vi "Logger_SendMessage.vi"(8 "error in (no error)":errorcluster caption="错误输入（无错误）", 9 "LoggerMessage":string, 10 "LoggerCode":i32=-1, 11 "LoggerKind":enum16{"软件上传日志", "软件其他日志", "软件错误日志", "软件监控日志"}(ring)=enum."软件监控日志") -> (0 "error out":errorcluster caption="错误输出")   [LabVIEW 2019, in "Logger.lvclass"]
uses:
  <userlib>/Logger/Logger.lvclass
  <userlib>/Logger/Ctls/LoggerMessage.ctl
  <userlib>/Logger/Logger.lvclass/Logger.ctl
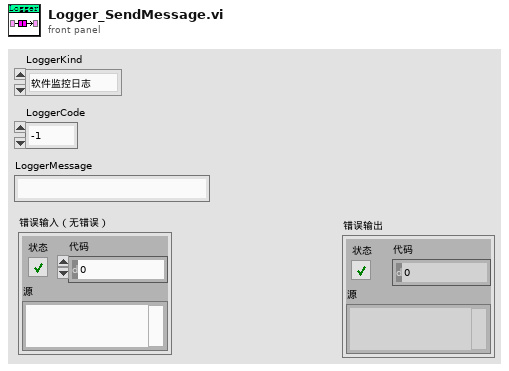
[diagram p1: front panel]
types:
  T1 = typedef "Logger.lvclass/LoggerMessage.ctl" = cluster{"LoggerKind":enum16{"软件上传日志", "软件其他日志", "软件错误日志", "软件监控日志"}, "LoggerMessage":string, "LoggerCode":i32, "LoggerCallChain":string, "LoggerTime":string}
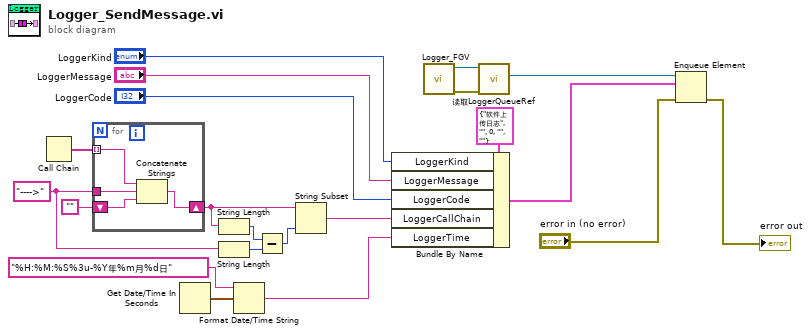
[diagram p0: block diagram]
diagram:
  w4 = "---->"
  n1 = Call Chain() -> (call chain=w17:string[])
  n2 = for {
    tunnel: w17 -> [w25] mode=indexing
    shift-right: [w22] -> w5
    shift-left: "" -> [w23]
    tunnel: w4 -> [w24]
    n3 = Concatenate Strings(w25, w24, w23) -> (w22:string)
  }
  n4 = Get Date/Time In Seconds() -> (seconds since 1Jan1904=w9:timestamp)
  n5 = String Length(string=w5) -> (length=w2:i32)
  n6 = String Length(string=w4) -> (length=w3:i32)
  n7 = Format Date/Time String(time format string (%c)="%H:%M:%S%3u-%Y年%m月%d日" ("时间格式字符串(%c)"), seconds (now)=w9) -> (date/time string=w7:string)  [unwired: 1 in]
  n8 = Subtract(x=w2, y=w3) -> (x-y=w1:i32)
  n9 = String Subset(string=w5, length (rest)=w1) -> (substring=w6:string)  [unwired: 1 in]
  n10 = Bundle By Name(cluster=T1 {"LoggerKind"=enum."软件上传日志", "LoggerMessage"="", "LoggerCode"=0, "LoggerCallChain"="", "LoggerTime"=""} ("元素"), "LoggerKind"="LoggerKind", "LoggerMessage"="LoggerMessage", "LoggerCode"="LoggerCode", "LoggerCallChain"=w6, "LoggerTime"=w7) -> (w20:T1)
  n11 = call <userlib>:"Logger_FGV.vi"() -> ("error out"=w11:errorcluster, "Logger 输出"=w12:refnum<class "Logger.lvclass">)  [unwired: 10 in]
  n12 = call "读取LoggerQueueRef.vi"("error in (no error)"=w11, "Logger输入"=w12) -> ("LoggerQueueRef"=w10:refnum<queue>)  [unwired: 7 in, 2 out]
  n13 = Enqueue Element(queue=w10, element=w20, error in (no error)="error in (no error)") -> (error out=→"error out":errorcluster)  [unwired: 1 in, 2 out]
